vi "Plot Global Rectangles.vi"(7 "Text Color (red)":u32(colorbox)=16711680, 8 "error in":errorcluster, 10 "Global Rectangles Array":T2(array[cluster]), 11 "Image In":T1) -> (0 "error out":errorcluster, 3 "Image Out":T1)   [LabVIEW 2012, in "Visual Analyser.lvlib"]
uses:
  Visual Analyser.lvlib
  <vilib>/vision/Image Controls.llb/IMAQ Image.ctl
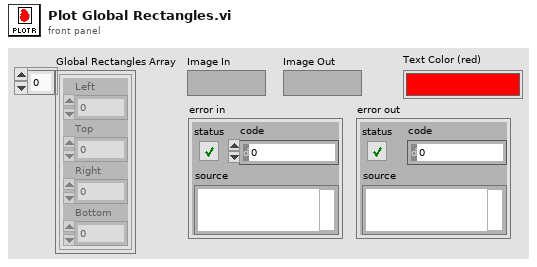
[diagram p1: front panel]
types:
  T1 = typedef "IMAQ Image.ctl" = refnum<image>
  T2 = cluster{"Left":dbl, "Top":dbl, "Right":dbl, "Bottom":dbl}[]
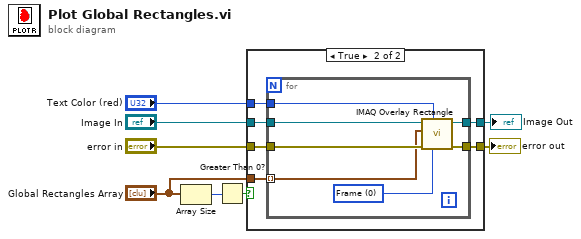
[diagram p0: block diagram]
diagram:
  n1 = Array Size(array="Global Rectangles Array") -> (size(s)=w8:i32)
  n2 = Greater Than 0?(x=w8) -> (x > 0?=w7:bool)
  n3 = case shown="True" w7 {
    tunnel: [w9 w16] -> w3
    tunnel: "Text Color (red)" -> [_ w15]
    tunnel: "Image In" -> [w10 w14]
    tunnel: [w10 w13] -> w5
    tunnel: "error in" -> [w9 w12]
    tunnel: "Global Rectangles Array" -> [_ w11]
    frame False {
    }
    frame True {
      n4 = for {
        tunnel: w12 -> [w20]
        tunnel: [w23] -> w16
        tunnel: [w22] -> w13
        tunnel: w14 -> [w21]
        tunnel: w15 -> [w19]
        tunnel: w11 -> [w17] mode=indexing
        w18 = u32 0 items=["Frame", "Fill", "Highlight"] ("Drawing Mode (Frame)")
        n5 = call "IMAQ Overlay Rectangle"("Color"=w19, "error in (no error)"=w20, "Drawing Mode (Frame)"=w18, "Rectangle"=w17, "Image"=w21) -> ("error out"=w23:errorcluster, "Image Out"=w22:T1)  [unwired: 5 in]
      }
    }
  }
  "error out" <- w3
  "Image Out" <- w5
